vi "Extract Window Origin and Size.vi"(11 "window rect":T1) -> (1 "window size":cluster{"width":i16, "height":i16}, 3 "window origin":cluster{"left":i16, "top":i16})   [LabVIEW 2020, in "MacroAssert.lvlib" / "WINUTIL.lvlib"]
doc: "This VI will extract the size and origin of a window using the window rectangle as an input. This information is useful when moving or resizing a window."
uses:
  WINUTIL.lvlib
  Window Rectangle.ctl
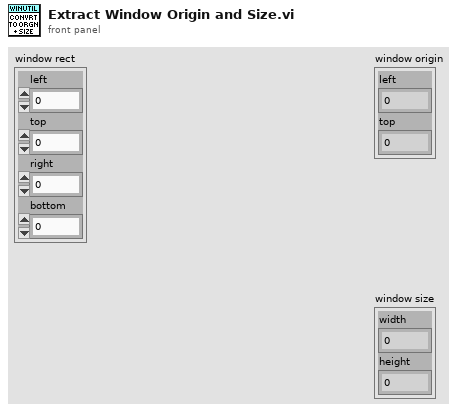
[diagram p1: front panel]
types:
  T1 = typedef "MacroAssert.lvlib/WINUTIL.lvlib/Window Rectangle.ctl" = cluster{"left":i16, "top":i16, "right":i16, "bottom":i16}
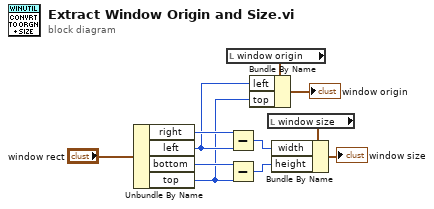
[diagram p0: block diagram]
diagram:
  n1 = Unbundle By Name("window rect") -> ("right"=w10:i16, "left"=w2:i16, "bottom"=w9:i16, "top"=w1:i16)
  n2 = local read "window origin"() -> (w4:cluster{"left":i16, "top":i16})
  n3 = Subtract(x=w10, y=w2) -> (x-y=w6:i16)
  n4 = Subtract(x=w9, y=w1) -> (x-y=w7:i16)
  n5 = Bundle By Name(cluster=w4, "left"=w2, "top"=w1) -> (→"window origin":cluster{"left":i16, "top":i16})
  n6 = local read "window size"() -> (w5:cluster{"width":i16, "height":i16})
  n7 = Bundle By Name(cluster=w5, "width"=w6, "height"=w7) -> (→"window size":cluster{"width":i16, "height":i16})
